vi "rqp_Save Spectrogramme Data.vi"(4 "Show in Debugger?":bool=TRUE, 6 "Message Priority":T1=enum."Normal", 7 "Caller in":refnum<class "Worker.lvclass">, 8 "error in":errorcluster, 10 "Data in":T2={"Save SpecTG"=FALSE, "Paramètres longueur d'onde"={"N"=2068, "lambda_0"=200.6310762, "lambda_c"=674.8888701568728, "d_lambda"=0.44435503366880597}, "FROG Trace"=[], "pas (um)"=0.0, "Nbre de scans"=0, "WL Values"=[]}, 11 "File manipulate in":refnum<class "File manipulate.lvclass">) -> (0 "error out":errorcluster, 3 "dup File manipulate out":refnum<class "File manipulate.lvclass">, 5 "dup Caller out":refnum<class "Worker.lvclass">)   [LabVIEW 2024, in "File manipulate.lvclass"]
doc: "This VI sends a <b>Public API Request</b> message to an MHL case of the Worker that owns this VI.\n---\nSauvegarde les données du spectrogramme dans un fichier"
uses:
  File manipulate.lvclass
  C:/Program Files (x86)/National Instruments/LabVIEW 2024/vi.lib/addons/_Workers/Library/Classes/Worker/Worker.lvclass
  <vilib>/addons/_Workers/Library/Classes/Worker/Worker.lvclass
  rqp_Save Spectrogramme Data.ctl
  <vilib>/addons/_Workers/Library/Classes/Message/Priority.ctl
  <vilib>/addons/_Workers/Library/Case Label.ctl
  <vilib>/addons/_Workers/Library/Classes/Message Queue/Message Queue.lvclass
  <vilib>/addons/_Workers/Library/Workers.lvlib
  <vilib>/addons/_Workers/Library/Classes/Message/Message.lvclass
  UI SmarAct/UI SmarAct.lvclass
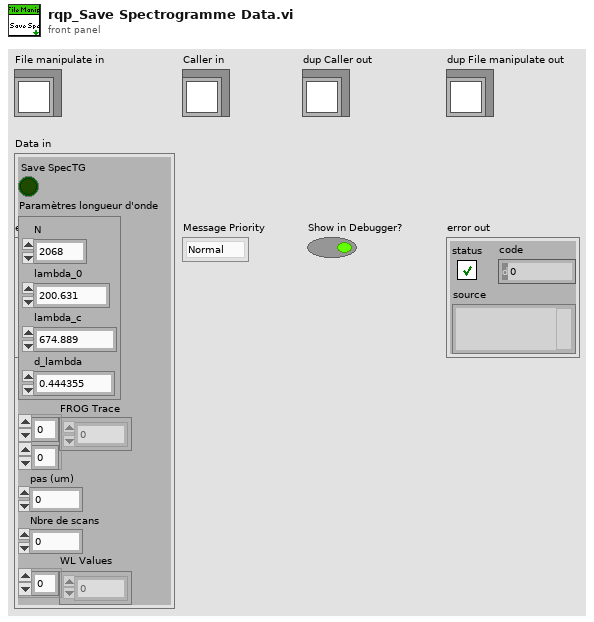
[diagram p1: front panel]
types:
  T1 = typedef "Workers.lvlib/Message.lvclass/Priority.ctl" = enum16{"Low", "Normal", "High"}
  T2 = typedef "File manipulate.lvclass/rqp_Save Spectrogramme Data.ctl" = cluster{"Save SpecTG":bool, "Paramètres longueur d'onde":T3, "FROG Trace":dbl[][], "pas (um)":dbl, "Nbre de scans":i32, "WL Values":dbl[]}
  T3 = typedef "UI SmarAct.lvclass/Paramètres longueur d'onde.ctl" = cluster{"N":i32, "lambda_0":dbl, "lambda_c":dbl, "d_lambda":dbl}
  T4 = typedef "Workers.lvlib/Case Label.ctl" = string
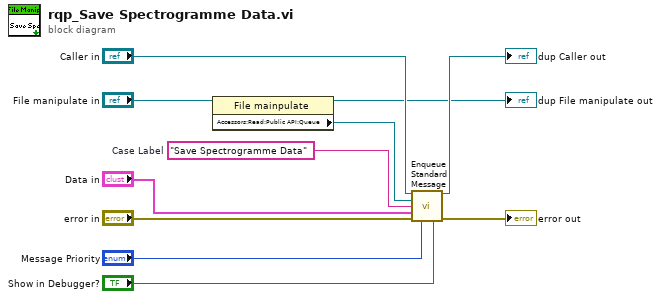
[diagram p0: block diagram]
diagram:
  w1 = T4 "Save Spectrogramme Data"  # Case Label
  n1 = property class="File mainpulate"(reference="File manipulate in") -> (reference out=→"dup File manipulate out":refnum<class "File manipulate.lvclass">, "Accessors:Read:Public API:Queue"=w2:refnum<class "Message Queue.lvclass">)  [unwired: 1 in, 1 out]
  n2 = call-dynamic "Enqueue Standard Message.vi"("Worker"="Caller in", "Message Queue"=w2, "Case Label"=w1, "Data"="Data in", "error in (no error)"="error in", "Priority (Normal)"="Message Priority", "Send Message to Debugger? (T)"="Show in Debugger?") -> ("dup Worker out"=→"dup Caller out":refnum<class "Worker.lvclass">, "error out"=→"error out":errorcluster)  [unwired: 7 in]
